vi "ServiceHostWait.vi"(2 "node":string, 3 "Topic":string="/junk", 4 "Type":string, 6 "error in":errorcluster) -> (0 "Request":string, 5 "Service ROS info out":T1={"topic port"=0, "Node"="", "topic"="", "type"="", "node port"=0, "error "={"status"=FALSE, "code"=0, "source"=""}, "Direction"=enum."Node", "Update (ms)"=1, "FIFO size"=1})   [LabVIEW 2016]
doc: "Starts a service host and returns an error if no request for that service has been made."
uses:
  ROS/Code/SubVIs/_ROSControl.ctl
  ROS/Code/SubVIs/_ROSDirection.ctl
  ROS/Code/Console/Servers/ServerSubs/TopicDef.ctl
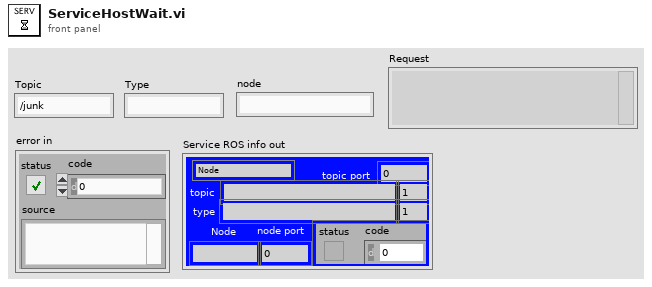
[diagram p1: front panel]
types:
  T1 = typedef "_ROSControl.ctl" = cluster{"topic port":u16, "Node":string, "topic":string, "type":string, "node port":u16, "error ":errorcluster, "Direction":T2, "Update (ms)":u16, "FIFO size":u16}
  T2 = typedef "_ROSDirection.ctl" = enum16{"Node", "Publisher", "Subscriber", "ServiceClient", "ServiceProvider"}
  T3 = typedef "TopicDef.ctl" = cluster{"Topic":string, "Type":string, "Action":T2, "Update (ms)":u16, "queue size":u16}
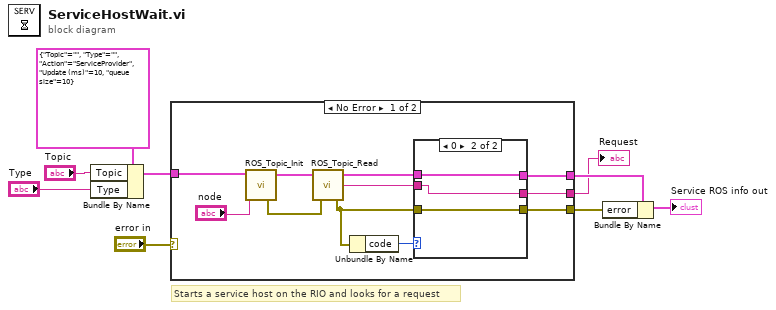
[diagram p0: block diagram]
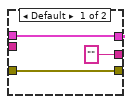
[diagram p2: hidden frame]
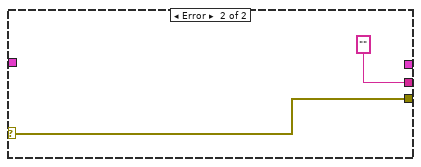
[diagram p3: hidden frame]
diagram:
  # "Starts a service host on the RIO and looks for a request"
  n1 = Bundle By Name(cluster=T3 {"Topic"="", "Type"="", "Action"=enum."ServiceProvider", "Update (ms)"=10, "queue size"=10} ("Definitions"), "Topic"="Topic", "Type"="Type") -> (w7:T3)
  n2 = case shown="No Error" "error in" {
    selector: "error in" -> [_ w28]
    tunnel: w7 -> [w19 _]
    tunnel: [w16 w28] -> w5
    tunnel: [w12 _] -> w4
    tunnel: [w10 "" ("msg out")] -> w2
    frame No Error {
      n3 = call "ROS_Topic_Init.vi"("Definitions"=w19, "node"="node") -> ("ROS out"=w18:T1, "error out"=w17:errorcluster)  [unwired: 1 in]
      n4 = call "ROS_Topic_Read.vi"("error in (no error)"=w17, "ROS in"=w18) -> ("error out"=w15:errorcluster, "Reply"=w14:string, "ROS out"=w13:T1)  [unwired: 1 in]
      n5 = Unbundle By Name(w15) -> ("code"=w11:i32)
      n6 = case shown="0" w11 {
        tunnel: [w22 w24] -> w16
        tunnel: w15 -> [w22 w24]
        tunnel: w14 -> [_ w25]
        tunnel: w13 -> [w23 w26]
        tunnel: [w23 w26] -> w12
        tunnel: ["" ("string") w25] -> w10
        frame Default {
        }
        frame 0 {
        }
      }
    }
    frame Error {
    }
  }
  "Request" <- w2
  n7 = Bundle By Name(cluster=w4, "error"=w5) -> (→"Service ROS info out":T1)
